vi "Async Initialize.vi"(8 "error in (no error)":errorcluster, 10 "Bus Settings":T1={"Name"="", "Overrides?"=FALSE, "XNET Refs"={"Incoming"="", "Outgoing"=""}, "Port Info"={"Port"="", "Baud Rate"=0, "Termination"=0, "CAN I/O Mode"=0, "FD Baud Rate"=500000, "Priority"=100, "FD ISO Mode"=0}, "Frames"=variant(cluster{"Convert Session":refnum<k21>, "ID":u32, "Length":i32, "Offset":i32}[] [])} {"Port Info"."FD ISO Mode" items=["ISO", "Non ISO", "ISO Legacy"]; "Port Info"."CAN I/O Mode" items=["CAN 2.0", "CAN FD", "CAN FD+BRS"]; "Port Info"."Termination" items=["Off", "On"]}, 11 "Process in":refnum<class "Process.lvclass">) -> (0 "error out":errorcluster, 2 "Execute":bool, 3 "Variables":T4={"Process Ref"=refnum, "Comm Ref"=refnum, "Bus Info"={"Name"="", "Overrides?"=FALSE, "XNET Refs"={"Incoming"="", "Outgoing"=""}, "Port Info"={"Port"="", "Baud Rate"=0, "Termination"=0, "CAN I/O Mode"=0, "FD Baud Rate"=500000, "Priority"=100, "FD ISO Mode"=0}, "Frames"=variant(cluster{"Convert Session":refnum<k21>, "ID":u32, "Length":i32, "Offset":i32}[] [])}, "Stream Refs"={"Addon"="", "Port"="", "Filter Ref"=refnum, "Default Filter"={"ID Filters"=[], "Direction Filter"=enum."Tx/Rx", "Type Filter"=enum."All"}, "Port Settings"={"Mode"=0, "Baud Rate"=0, "Termination"=0, "FD ISO Mode"=0, "FD Baud Rate"=0}}, "Data Refs"={"Port.Status"=refnum, "Frame.Enable"=refnum, "Frame.Signals"=refnum, "Frame.Overrides"=refnum, "Port.Enable"=refnum}} {"Stream Refs"."Port Settings"."FD ISO Mode" items=["ISO", "Non ISO", "ISO Legacy"]; "Stream Refs"."Port Settings"."Termination" items=["Off", "On"]; "Stream Refs"."Port Settings"."Mode" items=["CAN 2.0", "CAN FD", "CAN FD+BRS"]; "Bus Info"."Port Info"."FD ISO Mode" items=["ISO", "Non ISO", "ISO Legacy"]; "Bus Info"."Port Info"."CAN I/O Mode" items=["CAN 2.0", "CAN FD", "CAN FD+BRS"]; "Bus Info"."Port Info"."Termination" items=["Off", "On"]})   [LabVIEW 2019, in "Ghost Bus Addon Engine.lvlib"]
uses:
  Ghost Bus Addon Engine.lvlib
  Types/RT Async Engine Variables.ctl
  <vilib>/NI/NIVS Inline Async API/_VS Inline Async API/Process/Process.lvclass
  <vilib>/NI/NI VeriStand Addon Network Comm/Engine/VeriStand Comm.lvclass
  Types/RT Bus Settings.ctl
  Types/RT XNET Refs.ctl
  Addon Shared/Types/XNET Port Settings.ctl
  SubModules/CAN-Streaming-Support/Source/Addon/Addon Engine/Types/Engine Stream Refs.ctl
  SubModules/CAN-Streaming-Support/Source/Addon/Addon Shared/Types/Direction Filter.ctl
  SubModules/CAN-Streaming-Support/Source/Addon/Addon Shared/Types/Type Filter.ctl
  SubModules/CAN-Streaming-Support/Source/Addon/Addon Shared/Types/Filter Parameters.ctl
  SubModules/CAN-Streaming-Support/Source/Addon/Addon Engine/Types/Engine Stream Port Settings.ctl
  Types/RT Data Refs.ctl
  <vilib>/NI/NIVS Inline Async API/_Data Access Engine/Data Access Engine/Types/Write.DVR.ctl
  <vilib>/NI/NIVS Inline Async API/_Data Access Engine/Access Type Classes/Write/Write.lvclass
  <vilib>/NI/NIVS Inline Async API/_Data Access Engine/Data Access Engine/Types/Read.DVR.ctl
  <vilib>/NI/NIVS Inline Async API/_Data Access Engine/Access Type Classes/Read/Read.lvclass
  <vilib>/NI/NI VeriStand Addon Network Comm/Engine/VeriStand Comm.lvclass/VeriStand Comm.ctl
  <vilib>/NI/NIVS Inline Async API/_VS Inline Async API/Process/Process.lvclass/Process.ctl
  <vilib>/NI/NIVS Inline Async API/_VS Inline Async API/Process/Data Member Access/Read Data Access.vi
  <vilib>/NI/NIVS Inline Async API/_VS Inline Async API/Error Handling Process/SubVIs/Error.ConvertArray.vi
  Addon Shared/SubVIs/GUID Lookup.vi
  <vilib>/Utility/SystemLogging/Write to System Log.vi
  <vilib>/NI/AMC/Create Message Queue.vi
  <vilib>/NI/STM/Connection Manager/TCP/Advanced/TCP Initialize Connection Manager (By Reference).vi
  <vilib>/NI/NIVS Inline Async API/_Data Access Engine/Data Access Engine/Methods/Read.Lookup.vi
  <vilib>/NI/NIVS Inline Async API/_Data Access Engine/Data Access Engine/Methods/Write.Lookup.vi
  <vilib>/NI/NIVS Inline Async API/_Data Access Engine/Data Access Engine/Data Access Engine.lvclass
  SubModules/CAN-Streaming-Support/Source/Addon/Addon Shared/CAN Stream Support Shared.lvlib
  SubModules/CAN-Streaming-Support/Source/Addon/Addon Engine/CAN Stream Support Engine.lvlib
  <resource>/objmgr/xnet.rc
  Addon Shared/Ghost Bus Addon Shared.lvlib
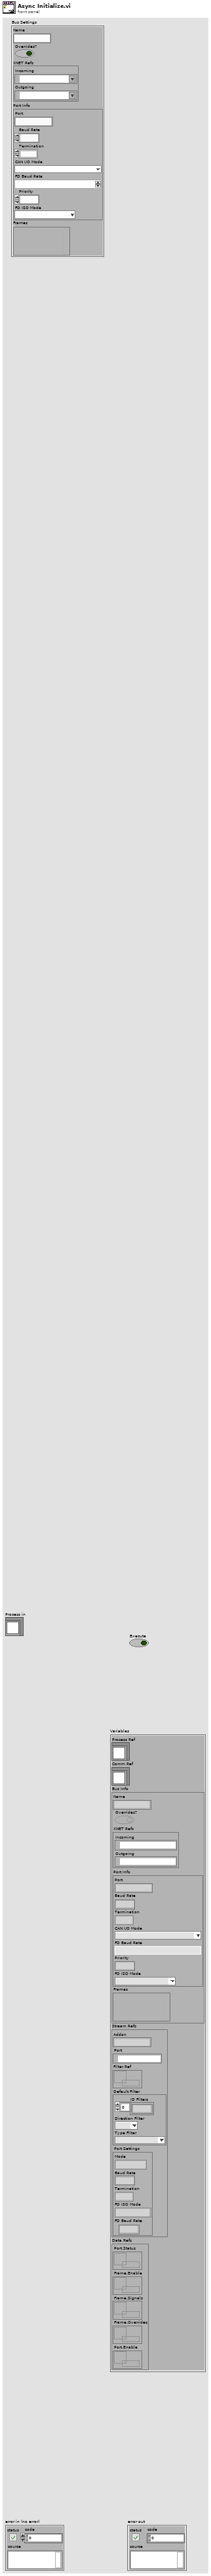
[diagram p1: front panel]
types:
  T1 = typedef "RT Bus Settings.ctl" = cluster{"Name":string, "Overrides?":bool, "XNET Refs":T2, "Port Info":T3, "Frames":variant}
  T2 = typedef "Ghost Bus Addon Engine.lvlib/RT XNET Refs.ctl" = cluster{"Incoming":refnum<k21>, "Outgoing":refnum<k21>}
  T3 = typedef "Ghost Bus Addon Shared.lvlib/XNET Port Settings.ctl" = cluster{"Port":string, "Baud Rate":u64, "Termination":u32, "CAN I/O Mode":u32, "FD Baud Rate":u64, "Priority":i32, "FD ISO Mode":u32}
  T4 = typedef "Ghost Bus Addon Engine.lvlib/RT Async Engine Variables.ctl" = cluster{"Process Ref":refnum<class "Process.lvclass">, "Comm Ref":refnum<class "VeriStand Comm.lvclass">, "Bus Info":T1, "Stream Refs":T5, "Data Refs":T10}
  T5 = typedef "CAN Stream Support Engine.lvlib/Engine Stream Refs.ctl" = cluster{"Addon":string, "Port":refnum<k21>, "Filter Ref":refnum<data-value>, "Default Filter":T6, "Port Settings":T9}
  T6 = typedef "CAN Stream Support Shared.lvlib/Filter Parameters.ctl" = cluster{"ID Filters":u32[], "Direction Filter":T7, "Type Filter":T8}
  T7 = typedef "CAN Stream Support Shared.lvlib/Direction Filter.ctl" = enum16{"Tx/Rx", "Rx", "Tx"}
  T8 = typedef "CAN Stream Support Shared.lvlib/Type Filter.ctl" = enum16{"All", "CAN Data", "CAN Remote", "CAN Bus Error", "CAN 2.0 Data", "CAN FD Data", "CAN FD+BRS Data", "J1939 Data", "Delay", "Log Trigger", "Start Trigger"}
  T9 = typedef "CAN Stream Support Engine.lvlib/Engine Stream Port Settings.ctl" = cluster{"Mode":u32, "Baud Rate":u64, "Termination":u32, "FD ISO Mode":u32, "FD Baud Rate":u64}
  T10 = typedef "Ghost Bus Addon Engine.lvlib/RT Data Refs.ctl" = cluster{"Port.Status":T11, "Frame.Enable":T12, "Frame.Signals":T12, "Frame.Overrides":T12, "Port.Enable":T12}
  T11 = typedef "Data Access Engine.lvlib/Data Access Engine.lvclass/Write.DVR.ctl" = refnum<data-value>
  T12 = typedef "Data Access Engine.lvlib/Data Access Engine.lvclass/Read.DVR.ctl" = refnum<data-value>
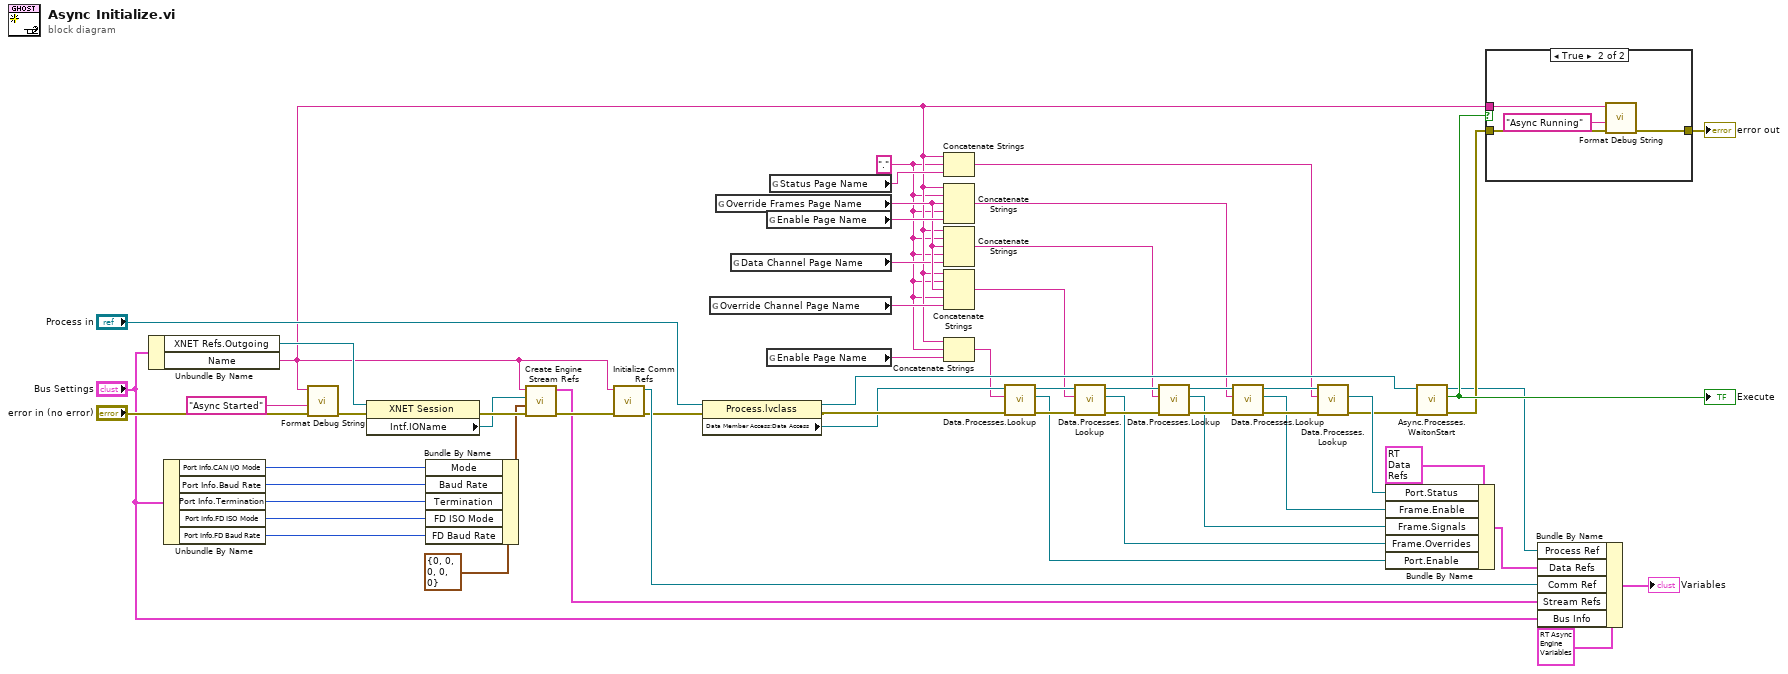
[diagram p0: block diagram]
diagram:
  w1 = "." ("string")
  n1 = Unbundle By Name("Bus Settings") -> ("XNET Refs.Outgoing"=w43:refnum<k21>, "Name"=w6:string)
  n2 = Unbundle By Name("Bus Settings") -> ("Port Info.CAN I/O Mode"=w37:u32, "Port Info.Baud Rate"=w34:u64, "Port Info.Termination"=w35:u32, "Port Info.FD ISO Mode"=w33:u32, "Port Info.FD Baud Rate"=w36:u64)
  n3 = call "Format Debug String.vi"("error in (no error)"="error in (no error)", "State"="Async Started", "Name"=w6) -> ("error out"=w45:errorcluster)  [unwired: 8 in]
  n4 = property class="XNET Session"(reference=w43, error in=w45) -> (error out=w44:errorcluster, "Intf.IOName"=w42:refnum<k21>)  [unwired: 1 out]
  n5 = Bundle By Name(cluster=T9 {"Mode"=0, "Baud Rate"=0, "Termination"=0, "FD ISO Mode"=0, "FD Baud Rate"=0} ("Port Settings"), "Mode"=w37, "Baud Rate"=w34, "Termination"=w35, "FD ISO Mode"=w33, "FD Baud Rate"=w36) -> (w38:T9)
  n6 = call "Create Engine Stream Refs.vi"("error in (no error)"=w44, "Port Settings"=w38, "Port"=w42, "Addon"=w6) -> ("error out"=w46:errorcluster, "Refs"=w41:T5)  [unwired: 6 in]
  n7 = call <vilib>:"Initialize Comm Refs.vi"("error in (no error)"=w46, "Name"=w6) -> ("error out"=w54:errorcluster, "Comm.lvclass"=w57:refnum<class "VeriStand Comm.lvclass">)  [unwired: 8 in]
  n8 = property class="Process.lvclass"(reference="Process in", error in=w54) -> (reference out=w48:refnum<class "Process.lvclass">, error out=w31:errorcluster, "Data Member Access:Data Access"=w30:refnum<class "Data Access Engine.lvclass">)
  n9 = global read "GUID Lookup.vi" "Override Channel Page Name"() -> (w8:string)
  n10 = global read "GUID Lookup.vi" "Override Frames Page Name"() -> (w10:string)
  n11 = global read "GUID Lookup.vi" "Data Channel Page Name"() -> (w9:string)
  n12 = global read "GUID Lookup.vi" "Enable Page Name"() -> (w11:string)
  n13 = global read "GUID Lookup.vi" "Enable Page Name"() -> (w13:string)
  n14 = global read "GUID Lookup.vi" "Status Page Name"() -> (w12:string)
  n15 = Concatenate Strings(w6, w1, w12) -> (w5:string)
  n16 = Concatenate Strings(w6, w1, w10, w1, w11) -> (w4:string)
  n17 = Concatenate Strings(w6, w1, w10, w1, w9) -> (w3:string)
  n18 = Concatenate Strings(w6, w1, w10, w1, w8) -> (w2:string)
  n19 = Concatenate Strings(w6, w1, w13) -> (w7:string)
  n20 = call-poly <vilib>:"Data.Processes.Lookup.vi"("error in (no error)"=w31, "Name"=w7, "Data Access API in"=w30) -> ("error out"=w28:errorcluster, "Ref"=w21:T12, "Data Access API out"=w29:refnum<class "Data Access Engine.lvclass">)  [unwired: 5 in, 1 out]
  n21 = call-poly <vilib>:"Data.Processes.Lookup.vi"("error in (no error)"=w28, "Name"=w2, "Data Access API in"=w29) -> ("error out"=w26:errorcluster, "Ref"=w20:T12, "Data Access API out"=w27:refnum<class "Data Access Engine.lvclass">)  [unwired: 5 in, 1 out]
  n22 = call-poly <vilib>:"Data.Processes.Lookup.vi"("error in (no error)"=w26, "Name"=w3, "Data Access API in"=w27) -> ("error out"=w24:errorcluster, "Ref"=w19:T12, "Data Access API out"=w25:refnum<class "Data Access Engine.lvclass">)  [unwired: 5 in, 1 out]
  n23 = call-poly <vilib>:"Data.Processes.Lookup.vi"("error in (no error)"=w24, "Name"=w4, "Data Access API in"=w25) -> ("error out"=w22:errorcluster, "Ref"=w18:T12, "Data Access API out"=w23:refnum<class "Data Access Engine.lvclass">)  [unwired: 5 in, 1 out]
  n24 = call-poly <vilib>:"Data.Processes.Lookup.vi"("error in (no error)"=w22, "Name"=w5, "Data Access API in"=w23) -> ("error out"=w15:errorcluster, "Ref"=w17:T11)  [unwired: 5 in, 2 out]
  n25 = Bundle By Name(cluster=T10 {"Port.Status"=refnum, "Frame.Enable"=refnum, "Frame.Signals"=refnum, "Frame.Overrides"=refnum, "Port.Enable"=refnum}, "Port.Status"=w17, "Frame.Enable"=w18, "Frame.Signals"=w19, "Frame.Overrides"=w20, "Port.Enable"=w21) -> (w14:T10)
  n26 = call <vilib>:"Async.Processes.WaitonStart.vi"("error in (no error)"=w15, "Process"=w48) -> ("error out"=w51:errorcluster, "Execute"=w53:bool, "Process out"=w32:refnum<class "Process.lvclass">)  [unwired: 7 in]
  "Execute" <- w53
  n27 = case shown="True" w53 {
    tunnel: w51 -> [w58 w61]
    tunnel: [w58 w60] -> w52
    tunnel: w6 -> [_ w59]
    frame False {
    }
    frame True {
      n28 = call "Format Debug String.vi"("error in (no error)"=w61, "State"="Async Running", "Name"=w59) -> ("error out"=w60:errorcluster)  [unwired: 8 in]
    }
  }
  "error out" <- w52
  n29 = Bundle By Name(cluster=T4 {"Process Ref"=refnum, "Comm Ref"=refnum, "Bus Info"={"Name"="", "Overrides?"=FALSE, "XNET Refs"={"Incoming"="", "Outgoing"=""}, "Port Info"={"Port"="", "Baud Rate"=0, "Termination"=0, "CAN I/O Mode"=0, "FD Baud Rate"=500000, "Priority"=100, "FD ISO Mode"=0}, "Frames"=variant(cluster{"Convert Session":refnum<k21>, "ID":u32, "Length":i32, "Offset":i32}[] [])}, "Stream Refs"={"Addon"="", "Port"="", "Filter Ref"=refnum, "Default Filter"={"ID Filters"=[], "Direction Filter"=enum."Tx/Rx", "Type Filter"=enum."All"}, "Port Settings"={"Mode"=0, "Baud Rate"=0, "Termination"=0, "FD ISO Mode"=0, "FD Baud Rate"=0}}, "Data Refs"={"Port.Status"=refnum, "Frame.Enable"=refnum, "Frame.Signals"=refnum, "Frame.Overrides"=refnum, "Port.Enable"=refnum}}, "Process Ref"=w32, "Data Refs"=w14, "Comm Ref"=w57, "Stream Refs"=w41, "Bus Info"="Bus Settings") -> (→"Variables":T4)
